vi "INTELLIFAUCET Flow Set.vi"(0 "VISA Refnum in":refnum<visa-resource-name>, 1 "TEMP,FLOW":T2=enum."FLOW", 2 "Use Proportion Valve":bool, 3 "Use General Conversion":bool, 5 "uA Set":i32, 9 "Temp/GPM Target":dbl=58.0 format="%#_13g", 11 "error in (no error)":errorcluster, 12 "Debug":bool, 13 "milliseconds to wait":u32=100, 14 "Refnum in":T1) -> (4 "VISA Refnum out":refnum<visa-resource-name>, 6 "Valve % Open":dbl, 10 "uA Output":i32, 15 "error out":errorcluster)   [LabVIEW 2016]
uses:
  Type Definitions/INTELLIFAUCT Temp Flow.ctl
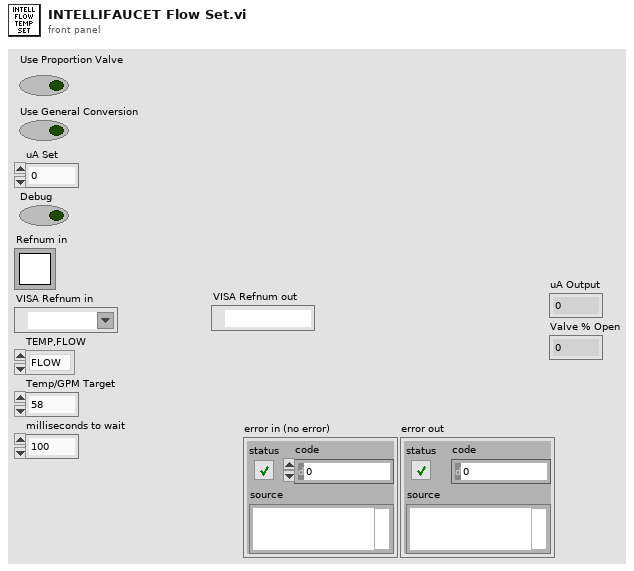
[diagram p1: front panel]
types:
  T1 = typedef "Semaphore RefNum" = refnum<k1>
  T2 = typedef "INTELLIFAUCT Temp Flow.ctl" = enum8{"TEMP", "FLOW"}
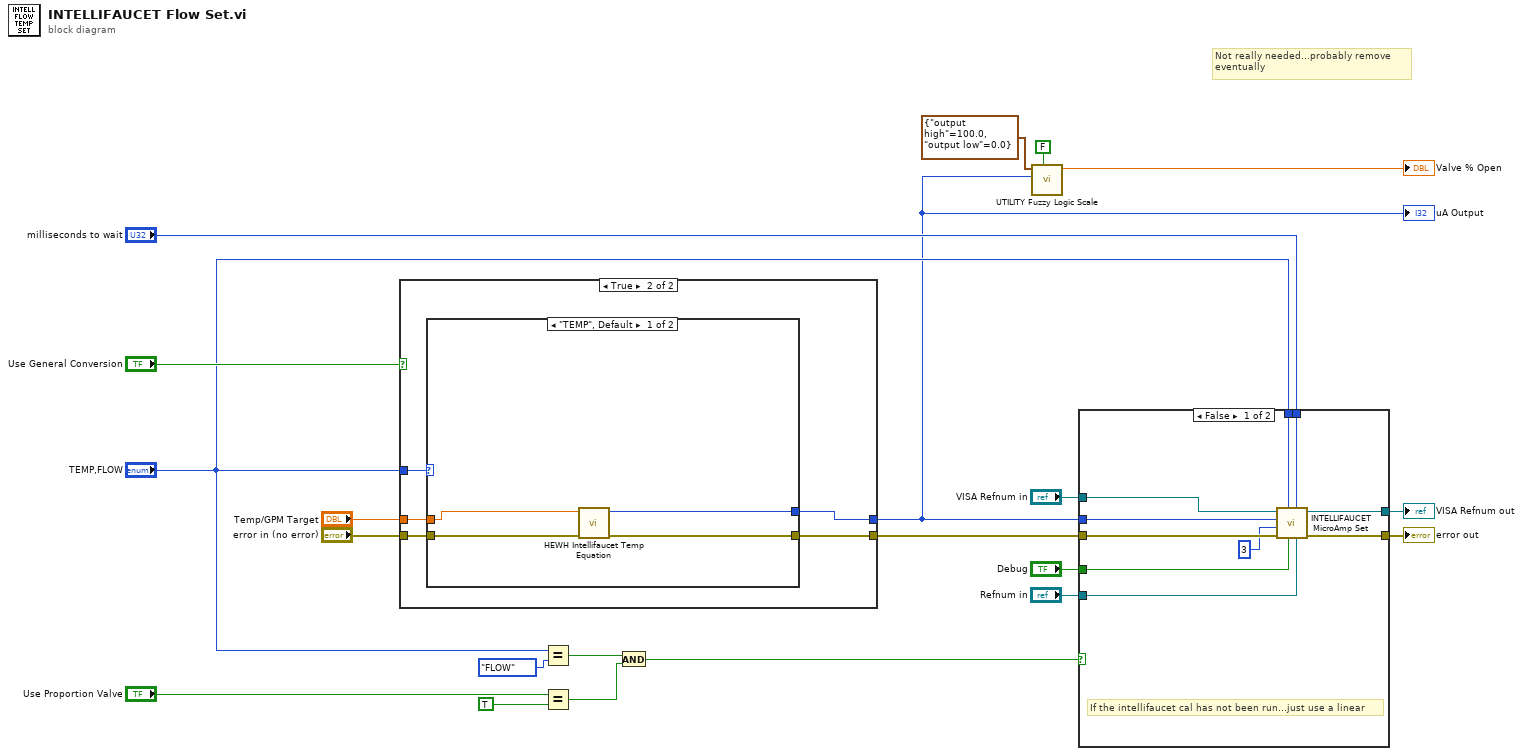
[diagram p0: block diagram]
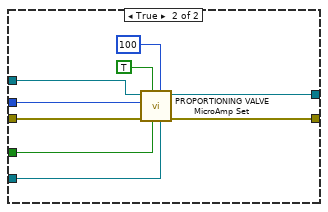
[diagram p2: hidden frame]
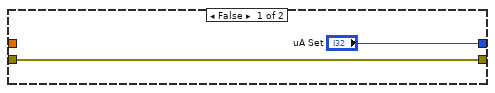
[diagram p3: hidden frame]
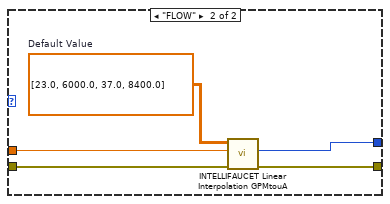
[diagram p4: hidden frame]
diagram:
  # "Not really needed...probably remove \neventually"
  n1 = case shown="True" "Use General Conversion" {
    tunnel: "error in (no error)" -> [w23 w28]
    tunnel: "Temp/GPM Target" -> [_ w27]
    tunnel: [w23 w26] -> w16
    tunnel: "TEMP,FLOW" -> [_ w24]
    tunnel: ["uA Set" w25] -> w2
    frame False {
    }
    frame True {
      n2 = case shown="\"TEMP\", Default" w24 {
        tunnel: w28 -> [w30 w37]
        tunnel: w27 -> [w32 w36]
        tunnel: [w29 w35] -> w26
        tunnel: [w31 w34] -> w25
        frame "TEMP", Default {
          n3 = call "HEWH Intellifaucet Temp Equation.vi"("Error In"=w30, "Temp/GPM Target"=w32) -> ("Error Out"=w29:errorcluster, "Temp uA"=w31:i32)  [unwired: 8 in]
        }
        frame "FLOW" {
          w33 = dbl[][] [[23.0, 6000.0], [37.0, 8400.0]]  # Default Value
          n4 = call "INTELLIFAUCET Linear Interpolation GPMtouA.vi"("Error In"=w37, "Target"=w36, "Interpolation Table(Xs,Ys)"=w33) -> ("Error Out"=w35:errorcluster, "uA Output"=w34:i32)  [unwired: 7 in]
        }
      }
    }
  }
  "uA Output" <- w2
  n5 = Equal?(x="TEMP,FLOW", y=INTELLIFAUCT_Temp_Flow."FLOW") -> (x = y?=w7:bool)
  n6 = Equal?(x="Use Proportion Valve", y=TRUE) -> (x = y?=w6:bool)
  n7 = And(x=w7, y=w6) -> (x .and. y?=w5:bool)
  n8 = call "UTILITY Fuzzy Logic Scale.vi"("Convert to MicroAmp (T), Standard Output (F)"=FALSE, "input variable"=w2, "output range"=cluster{"output high":dbl, "output low":dbl} {"output high"=100.0, "output low"=0.0}) -> ("MicroAmp"=→"Valve % Open":dbl)  [unwired: 7 in, 1 out]
  n9 = case shown="False" w5 {
    tunnel: "VISA Refnum in" -> [w47 w53]
    tunnel: [w46 w52] -> w20
    tunnel: [w45 w55] -> w19
    tunnel: w16 -> [w44 w54]
    tunnel: "TEMP,FLOW" -> [w43 _]
    tunnel: "Debug" -> [w42 w48]
    tunnel: "Refnum in" -> [w41 w49]
    tunnel: w2 -> [w39 w50]
    tunnel: "milliseconds to wait" -> [w38 _]
    frame False {
      # "If the intellifaucet cal has not been run...just use a linear"
      n10 = call "INTELLIFAUCET MicroAmp Set.vi"("Refnum in"=w41, "milliseconds to wait"=w38, "Debug"=w42, "TEMP,FLOW"=w43, "error in (no error)"=w44, "# of Retries"=3, "MicroAmp"=w39, "VISA Refnum in"=w47) -> ("error out"=w45:errorcluster, "VISA Refnum out"=w46:refnum<visa-resource-name>)  [unwired: 2 in]
    }
    frame True {
      n11 = call "PROPORTIONING VALVE MicroAmp Set.vi"("Refnum in"=w49, "milliseconds to wait"=u32 100, "Debug"=w48, "Use Micro Amp Set"=TRUE, "error in (no error)"=w54, "Target"=w50, "VISA Refnum in"=w53) -> ("error out"=w55:errorcluster, "VISA Refnum out"=w52:refnum<visa-resource-name>)  [unwired: 3 in]
    }
  }
  "VISA Refnum out" <- w20
  "error out" <- w19
